vi "Init_Instr.vi"(8 "error in (no error)":errorcluster caption="entrée d'erreur (pas d'erreur)", 11 "Class Instrument (Default) en entrée":refnum<class "Class Instrument (Default).lvclass">) -> (0 "error out":errorcluster caption="sortie d'erreur", 3 "Class Instrument (Default) en sortie":refnum<class "Class Instrument (Default).lvclass">)   [LabVIEW 2020, in "Library Instrument & Equipement.lvlib" / "Library Instruments.lvlib" / "Class Instrument (Default).lvclass"]
uses:
  Class Instrument (Default).lvclass
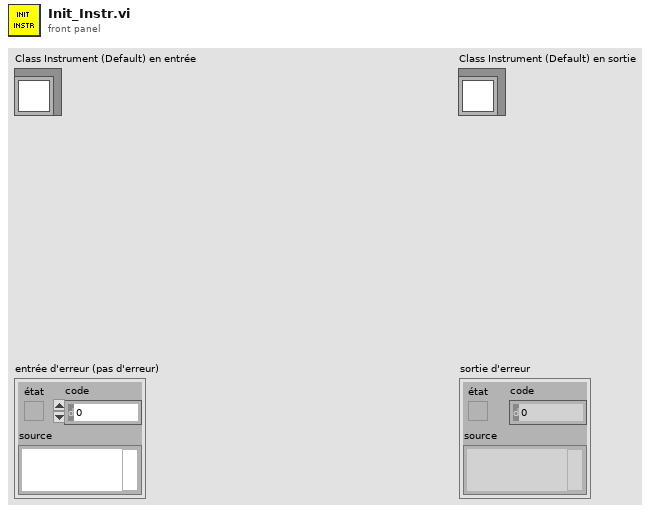
[diagram p1: front panel]
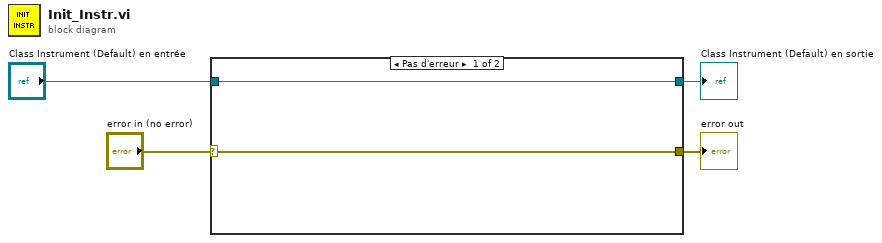
[diagram p0: block diagram]
diagram:
  n1 = case shown="Pas d'erreur" "error in (no error)" {
    selector: "error in (no error)" -> [w5 w8]
    tunnel: [w5 w8] -> w2
    tunnel: [w6 w7] -> w3
    tunnel: "Class Instrument (Default) en entrée" -> [w6 w7]
    frame No Error {
    }
    frame Error {
    }
  }
  "error out" <- w2
  "Class Instrument (Default) en sortie" <- w3
